vi "take from cube.vi"(10 "c2":i32, 11 "c1":i32) -> ()   [LabVIEW 2018]
uses:
  vision info 2.vi
panel:
  out "Numeric":i32
  in  "stop 2":bool
  in  "stop":bool
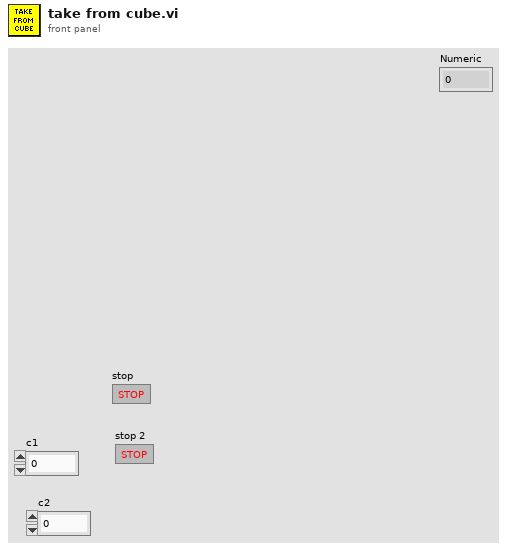
[diagram p1: front panel]
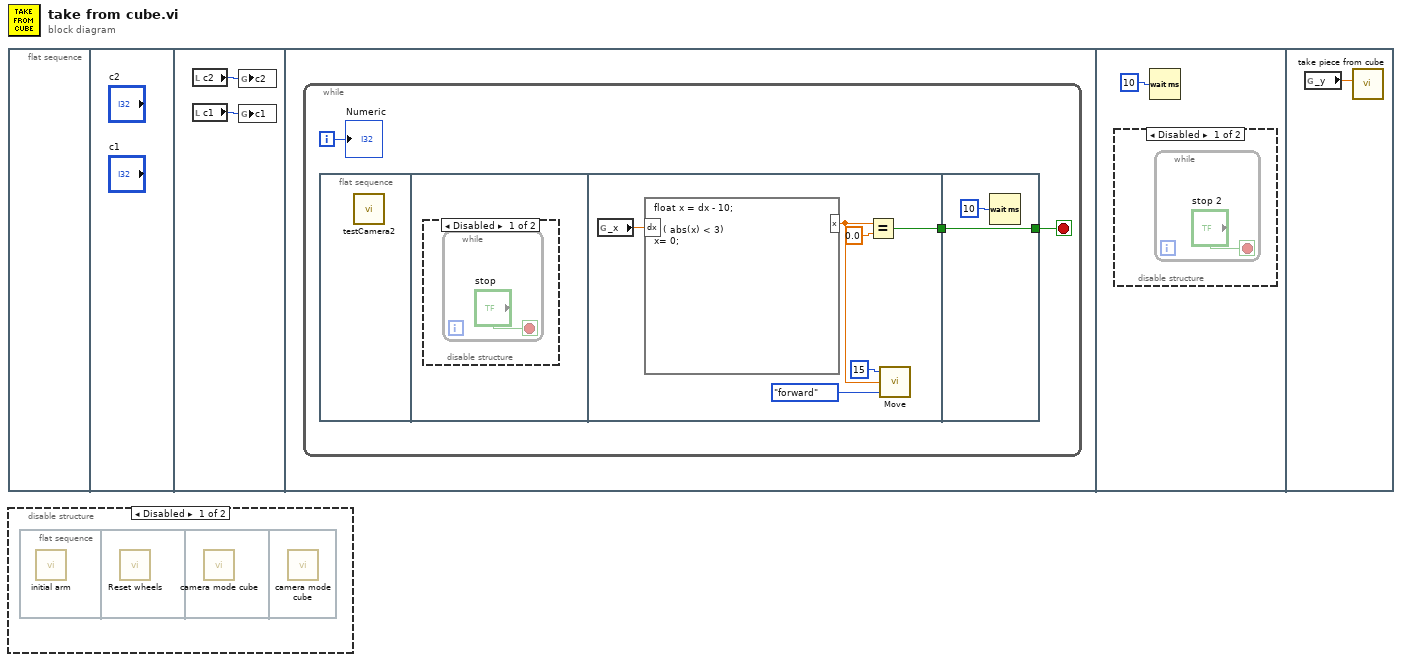
[diagram p0: block diagram]
diagram:
  n1 = flat-sequence {
    frame #0 {
    }
    frame #1 {
    }
    frame #2 {
      n2 = local read "c2"() -> (w1:i32)
      n3 = local read "c1"() -> (w2:i32)
      n4 = global write "vision info 2.vi" "c2"(w1) -> ()
      n5 = global write "vision info 2.vi" "c1"(w2) -> ()
    }
    frame #3 {
      n6 = while {
        i -> [w4]
        stop <- w5 stop-if-true
        n7 = flat-sequence {
          tunnel: [w7] -> w3
          tunnel: [w14] -> w5
          tunnel: w3 -> [w14]
          frame #0 {
            n8 = call "testCamera2.vi"() -> ()  [unwired: 12 in]
          }
          frame #1 {
            n9 = disable-structure shown="Disabled" {
              frame Disabled {
                n10 = while {
                  stop <- "stop" stop-if-true
                }
              }
              frame Enabled {
              }
            }
          }
          frame #2 {
            n11 = global read "vision info 2.vi" "_x"() -> (w12:dbl)
            n12 = formula code="float x = dx - 10;\n\nif ( abs(x) < 3)\nx= 0;"("dx"=w12) -> ("x"=w9:dbl)
            n13 = Equal?(x=w9, y=0.0) -> (x = y?=w7:bool)
            n14 = call "Move.vi"("Enum"=enum16{"forward", "backward", "left", "right"}."forward", "distance"=w9, "speed"=15) -> ()  [unwired: 1 in]
          }
          frame #3 {
            n15 = Wait (ms)(milliseconds to wait=u32 10) -> ()  [unwired: 1 out]
          }
        }
        "Numeric" <- w4
      }
    }
    frame #4 {
      n16 = disable-structure shown="Disabled" {
        frame Disabled {
          n17 = while {
            stop <- "stop 2" stop-if-true
          }
        }
        frame Enabled {
        }
      }
      n18 = Wait (ms)(milliseconds to wait=u32 10) -> ()  [unwired: 1 out]
    }
    frame #5 {
      n19 = global read "vision info 2.vi" "_y"() -> (w17:dbl)
      n20 = call "take piece from cube.vi"("y"=w17) -> ()  [unwired: 10 in]
    }
  }
  n21 = disable-structure shown="Disabled" {
    frame Disabled {
      n22 = flat-sequence {
        frame #0 {
          n23 = call "initial arm.vi"() -> ()  [unwired: 12 in]
        }
        frame #1 {
          n24 = call "Reset wheels.vi"() -> ()  [unwired: 12 in]
        }
        frame #2 {
          n25 = call "camera mode cube.vi"() -> ()  [unwired: 12 in]
        }
        frame #3 {
          n26 = call "camera mode cube.vi"() -> ()  [unwired: 12 in]
        }
      }
    }
    frame Enabled {
    }
  }
